vi "AskTurning.vi"(7 "Z Scan Parameters":T1={"Z Range"=1380.0, "Resolution"=5000.0, "Initial Direction"=enum."Up", "Focus Threshold"=0.1, "Ascent Constant"=0.1} {"Focus Threshold" min=0.0 max=1000.0 step=1.0 format="%#_2f"; "Ascent Constant" min=0.0 max=1000.0 step=1.0 format="%#_2f"; "Resolution" min=0.0 max=1.0 step=0.01 format="%_2g"; "Z Range" format="%_3g"}, 8 "error in (no error)":errorcluster, 9 "Edge Sherpness":sgl, 10 "Z":dbl, 11 "Function":enum16{"Turning?", "Reset"}(ring)) -> (0 "error out":errorcluster, 1 "Max Sharpness":sgl, 2 "Z @ Max Sharpness":dbl, 3 "Questions":T2)   [LabVIEW 2014]
uses:
  ZScan.ctl
  <vilib>/Analysis/NI_AALPro.lvlib
panel:
  out "dF":dbl(graph)
  out "Z":dbl(graph)
  out "dZ":dbl(graph)
  out "F":sgl(graph)
  # "LICENSED MATERIALS – PROPERTY OF IBM\nCopyright IBM Corp. 2016,\nALL RIGHTS RESERVED"
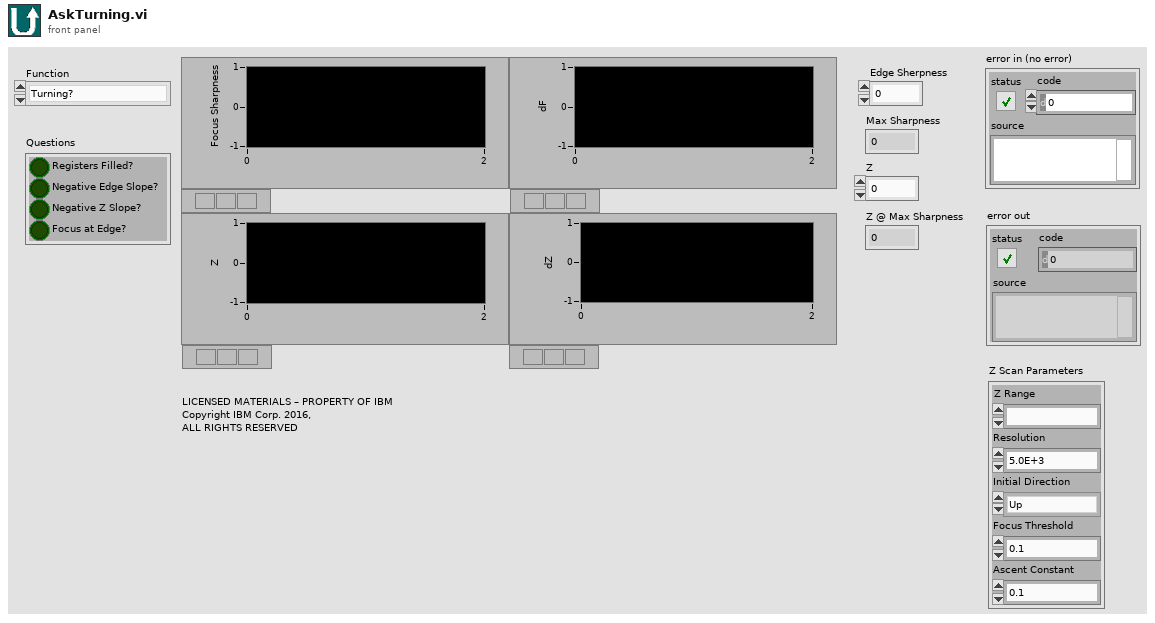
[diagram p1: front panel]
types:
  T1 = typedef "ZScan.ctl" = cluster{"Z Range":ext, "Resolution":dbl, "Initial Direction":enum16{"Up", "Down"}, "Focus Threshold":dbl, "Ascent Constant":dbl}
  T2 = cluster{"Registers Filled?":bool, "Negative Edge Slope?":bool, "Negative Z Slope?":bool, "Focus at Edge?":bool}
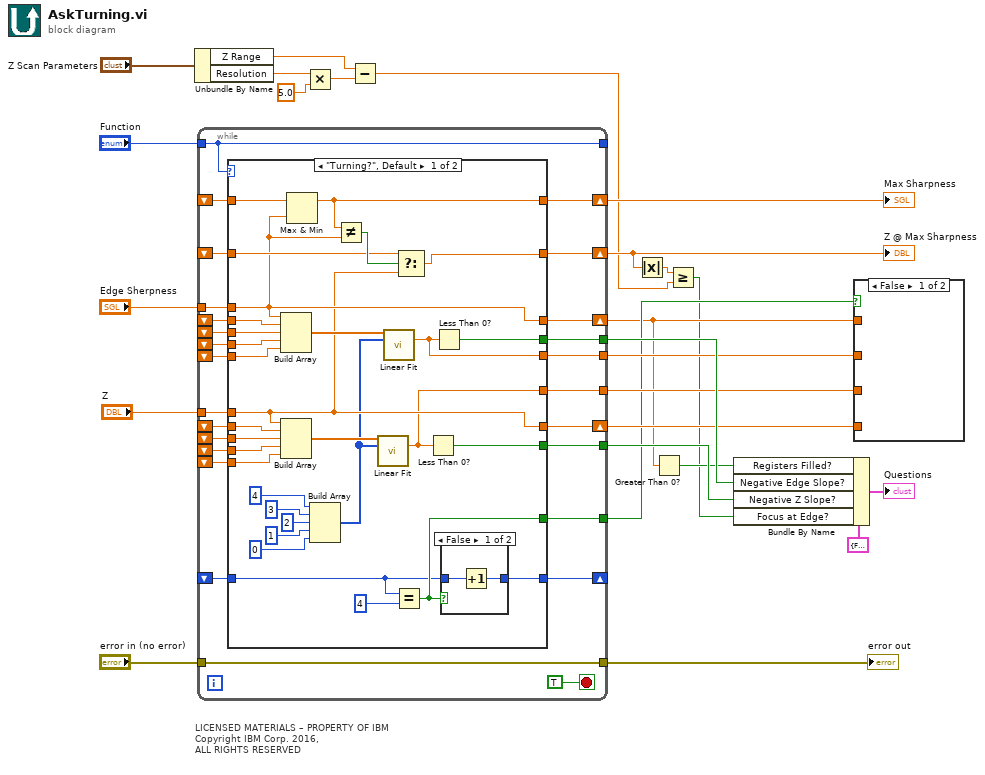
[diagram p0: block diagram]
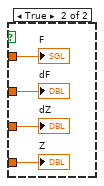
[diagram p2: hidden frame]
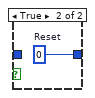
[diagram p3: hidden frame]
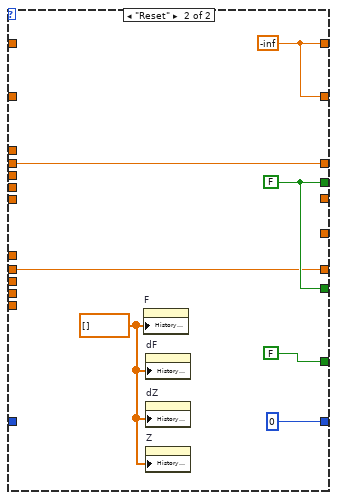
[diagram p4: hidden frame]
diagram:
  # "LICENSED MATERIALS – PROPERTY OF IBM\nCopyright IBM Corp. 2016,\nALL RIGHTS RESERVED"
  n1 = Unbundle By Name("Z Scan Parameters") -> ("Z Range"=w7:ext, "Resolution"=w5:dbl)
  n2 = while {
    tunnel: "Edge Sherpness" -> [w37]
    shift-right: [w36] -> w10
    shift-left: _ -> [w50]
    shift-right: [w51] -> _
    shift-left: _ -> [w45]
    shift-left: _ -> [w49]
    shift-left: _ -> [w48]
    shift-left: _ -> [w47]
    tunnel: [w44] -> w18
    tunnel: [w26] -> w12
    tunnel: "Function" -> [w27]
    tunnel: [w43] -> w23
    tunnel: "error in (no error)" -> [w43]
    shift-right: [w34] -> w17
    shift-left: _ -> [w42]
    tunnel: "Z" -> [w35]
    shift-left: _ -> [w41]
    shift-left: _ -> [w40]
    shift-left: _ -> [w39]
    tunnel: [w38] -> w16
    shift-right: [w31] -> w20
    shift-left: _ -> [w33]
    shift-right: [w30] -> w8
    shift-left: _ -> [w32]
    tunnel: [w29] -> w14
    tunnel: [w28] -> w13
    tunnel: [w27] -> _
    stop <- TRUE stop-if-true
    n3 = case shown="\"Turning?\", Default" w27 {
      tunnel: [w75 0] -> w51
      tunnel: w50 -> [w82 w89]
      tunnel: w49 -> [w81 _]
      tunnel: w48 -> [w80 _]
      tunnel: w47 -> [w79 _]
      tunnel: w37 -> [w63 _]
      tunnel: w45 -> [w52 _]
      tunnel: [w76 FALSE] -> w26
      tunnel: [w77 w90] -> w44
      tunnel: w35 -> [w62 _]
      tunnel: w42 -> [w71 w88]
      tunnel: w41 -> [w72 _]
      tunnel: w40 -> [w73 _]
      tunnel: w39 -> [w74 _]
      tunnel: [w69 w90] -> w38
      tunnel: [w63 w89] -> w36
      tunnel: [w62 w88] -> w34
      tunnel: w33 -> [w68 _]
      tunnel: w32 -> [w65 _]
      tunnel: [w66 w87] -> w31
      tunnel: [w64 w87] -> w30
      tunnel: [w61 _] -> w29
      tunnel: [w60 _] -> w28
      frame "Turning?", Default {
        n4 = Build Array(w63, w82, w81, w80, w79) -> (w78:sgl[])
        n5 = Build Array(w62, w71, w72, w73, w74) -> (w70:dbl[])
        n6 = Max & Min(x=w68, y=w63) -> (max(x,y)=w66:sgl)  [unwired: 1 out]
        n7 = Build Array(4 ("y"), 3 ("y"), 2 ("y"), 1 ("y"), 0 ("y")) -> (w54:i32[])
        n8 = Not Equal?(x=w66, y=w63) -> (x != y?=w67:bool)
        n9 = call <vilib>:"Linear Fit.vi"("Y"=w70, "X"=w54) -> ("slope"=w60:dbl)  [unwired: 9 in, 4 out]
        n10 = call <vilib>:"Linear Fit.vi"("Y"=w78, "X"=w54) -> ("slope"=w61:dbl)  [unwired: 9 in, 4 out]
        n11 = Equal?(x=w52, y=4) -> (x = y?=w76:bool)
        n12 = Select(t=w65, s=w67, f=w62) -> (s? t:f=w64:dbl)
        n13 = Less Than 0?(x=w60) -> (x < 0?=w69:bool)
        n14 = Less Than 0?(x=w61) -> (x < 0?=w77:bool)
        n15 = case shown="False" w76 {
          tunnel: [w83 w85] -> w75
          tunnel: w52 -> [w84 _]
          frame False {
            n16 = Increment(x=w84) -> (x+1=w83:i32)
          }
          frame True {
            w85 = 0  # Reset
          }
        }
      }
      frame "Reset" {
        w86 = sgl[] [] ("History Data")
        w87 = sgl -inf
        w90 = FALSE
        n17 = property on="F" class="WFChart (strict)"("History Data"=w86) -> ()  [unwired: 2 in, 2 out]
        n18 = property on="dF" class="WFChart (strict)"("History Data"=w86) -> ()  [unwired: 2 in, 2 out]
        n19 = property on="dZ" class="WFChart (strict)"("History Data"=w86) -> ()  [unwired: 2 in, 2 out]
        n20 = property on="Z" class="WFChart (strict)"("History Data"=w86) -> ()  [unwired: 2 in, 2 out]
      }
    }
  }
  "error out" <- w23
  "Max Sharpness" <- w20
  "Z @ Max Sharpness" <- w8
  n21 = Multiply(x=w5, y=5.0) -> (x*y=w3:dbl)
  n22 = Subtract(x=w7, y=w3) -> (x-y=w1:ext)
  n23 = Absolute Value(x=w8) -> (abs(x)=w2:dbl)
  n24 = Greater Than 0?(x=w10) -> (x > 0?=w11:bool)
  n25 = Greater Or Equal?(x=w2, y=w1) -> (x >= y?=w6:bool)
  n26 = Bundle By Name(cluster=T2 {"Registers Filled?"=FALSE, "Negative Edge Slope?"=FALSE, "Negative Z Slope?"=FALSE, "Focus at Edge?"=FALSE} ("Questions 2"), "Registers Filled?"=w11, "Negative Edge Slope?"=w18, "Negative Z Slope?"=w16, "Focus at Edge?"=w6) -> (→"Questions":T2)
  n27 = case shown="False" w12 {
    tunnel: w10 -> [_ w94]
    tunnel: w17 -> [_ w96]
    tunnel: w14 -> [_ w93]
    tunnel: w13 -> [_ w95]
    frame False {
    }
    frame True {
      "F" <- w94
      "dZ" <- w95
      "Z" <- w96
      "dF" <- w93
    }
  }
